vi "Process-error.vi"(8 "error in (no error)":errorcluster, 11 "Client in":T1) -> (0 "error out":errorcluster, 3 "Client out":T1)   [LabVIEW 2013, in "CameraVision.lvlib" / "CV-Client.lvclass"]
doc: "Processes any previously encountered error.\nThis function can process both the standard LabVIEW errors and the custom defined errors for this module.\nThe default implementation simply shows an error message box to the user and removes the error from the stream, without further affecting the program execution."
uses:
  CV-Client.lvclass
  Object-reference.ctl
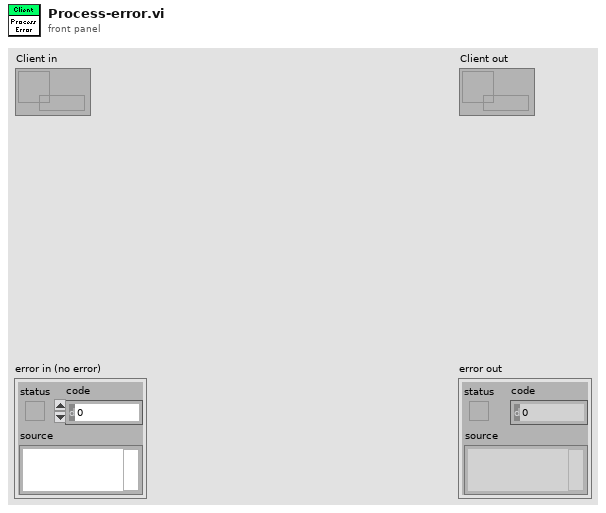
[diagram p1: front panel]
types:
  T1 = typedef "CameraVision.lvlib/CV-Client.lvclass/Object-reference.ctl" = refnum<data-value>
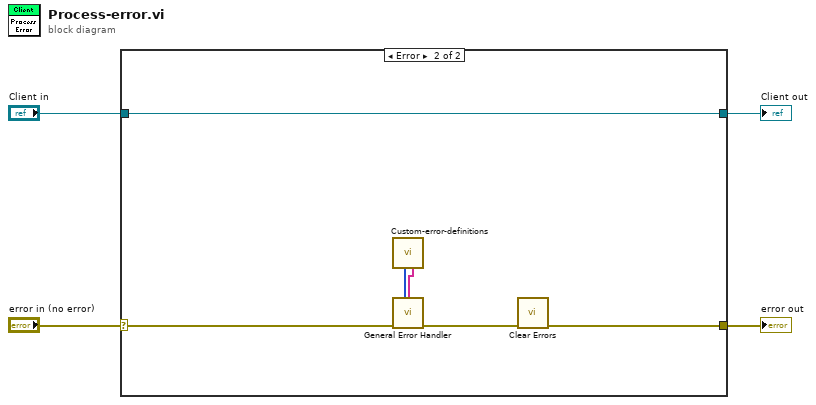
[diagram p0: block diagram]
diagram:
  n1 = case shown="Error" "error in (no error)" {
    selector: "error in (no error)" -> [w6 w12]
    tunnel: [w6 w7] -> w3
    tunnel: [w5 w11] -> w1
    tunnel: "Client in" -> [w5 w11]
    frame No Error {
    }
    frame Error {
      n2 = call "Custom-error-definitions.vi"() -> ("Descriptions"=w9:string[], "Error codes"=w10:i32[])  [unwired: 9 in, 1 out]
      n3 = call <vilib>:"General Error Handler.vi"("[user-defined codes]"=w10, "[user-defined descriptions]"=w9, "error in (no error)"=w12) -> ("error out"=w8:errorcluster)  [unwired: 8 in, 4 out]
      n4 = call <vilib>:"Clear Errors.vi"("error in (no error)"=w8) -> ("error out"=w7:errorcluster)  [unwired: 6 in]
    }
  }
  "error out" <- w3
  "Client out" <- w1
